vi "Konvolucio MCAN120803 Example_0002 ConnectTo.vi"() -> ()   [LabVIEW 2011]
uses:
  <instrlib>/Konvolucio MCAN120803/Types/AdapterItemType.ctl
  C:/Program Files/National Instruments/LabVIEW 2011/instr.lib/Konvolucio MCAN120803/Private/Konvolucio.MCAN120803.API.dll
  Private/Konvolucio.MCAN120803.API.dll
  <instrlib>/Konvolucio MCAN120803/Konvolucio MCAN120803.lvlib
panel:
  out "AdaptersOut":T1[](array[typedef])
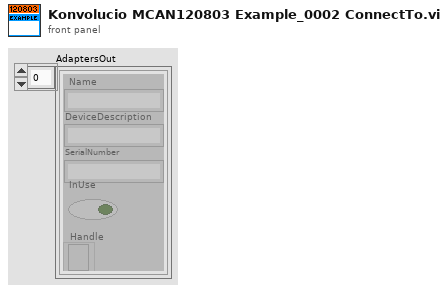
[diagram p1: front panel]
types:
  T1 = typedef "Konvolucio MCAN120803.lvlib/AdapterItemType.ctl" = cluster{"Name":string, "DeviceDescription":string, "SerialNumber":string, "InUse":bool, "Handle":refnum<k24>}
  T2 = typedef "Konvolucio MCAN120803.lvlib/CanHandleType.ctl" = cluster{"AdapterDevice":refnum<k24>}
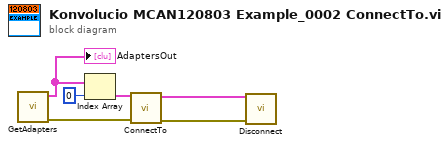
[diagram p0: block diagram]
diagram:
  n1 = call <instrlib>:"GetAdapters.vi"() -> ("error out"=w5:errorcluster, "AdaptersOut"=w4:T1[])  [unwired: 10 in]
  "AdaptersOut" <- w4
  n2 = Index Array(array=w4, index=0) -> (element=w3:T1)
  n3 = call <instrlib>:"ConnectTo.vi"("error in"=w5, "AdapterIn"=w3) -> ("error out"=w6:errorcluster, "CanHandleOut"=w2:T2)  [unwired: 8 in]
  n4 = call <instrlib>:"Disconnect.vi"("error in"=w6, "CanHandleIn"=w2) -> ()  [unwired: 9 in, 1 out]
